vi "Change Brightness.vi"(0 "Color In":u32(colorbox)=16711680, 7 "Multiplier":dbl=1.5, 11 "error in (no error)":errorcluster) -> (4 "Modified Color":u32(colorbox), 15 "error out":errorcluster)   [LabVIEW 2012, in "Picture Box Tools.lvlib"]
doc: "This VI lightens or darkens an image based on a multiplier value. Where the multiplier is X, for any given color this VI will return a color X times lighter. Values less than 1 for the multiplier will darken the color. Values greater than 1 will lighten the color.\n\nSee HSLToolsAdvancedExample.vi in the NI Example Finder for more information."
uses:
  Picture Box Tools.lvlib
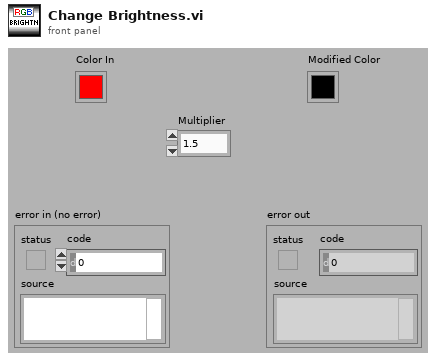
[diagram p1: front panel]
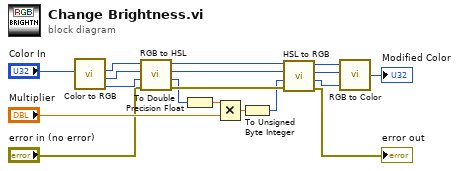
[diagram p0: block diagram]
diagram:
  n1 = call <vilib>:"Color to RGB.vi"("Color"="Color In") -> ("R"=w18:u8, "G"=w17:u8, "B"=w16:u8)  [unwired: 1 out]
  n2 = call <vilib>:"RGB to HSL.vi"("Error In"="error in (no error)", "Blue"=w16, "Green"=w17, "Red"=w18) -> ("Error Out"=w12:errorcluster, "Lum"=w8:u8, "Sat"=w10:u8, "Hue"=w11:u8)  [unwired: 4 out]
  n3 = To Double Precision Float(number=w8) -> (double precision float=w9:dbl)
  n4 = Multiply(x=w9, y="Multiplier") -> (x*y=w7:dbl)
  n5 = To Unsigned Byte Integer(number=w7) -> (unsigned 8bit integer=w6:u8)
  n6 = call <vilib>:"HSL to RGB.vi"("Error In"=w12, "Lum"=w6, "Sat"=w10, "Hue"=w11) -> ("Error Out"=→"error out":errorcluster, "Blue"=w13:u8, "Green"=w14:u8, "Red"=w15:u8)  [unwired: 4 out]
  n7 = call <vilib>:"RGB to Color.vi"("B"=w13, "G"=w14, "R"=w15) -> ("Color"=→"Modified Color":u32)
